vi "PersonnelFGV.vi"(7 "Actions":T1=enum."Read Personnel", 8 "error in (no error)":errorcluster, 9 "Data In":string, 10 "PUID":string) -> (0 "error out":errorcluster, 1 "Data Out":string)   [LabVIEW 2015]
uses:
  TypeDef/PersonnelActions.ctl
  TypeDef/PersonnelState.ctl
  LVClasses/Personnel/Personnel.lvclass
  LVClasses/Personnel/PersonnelType.ctl
  LVClasses/Personnel/Personnel.lvclass/Personnel.ctl
  LVClasses/Request/SummaryJsonCluster.ctl
  LVClasses/Personnel/Read Name.vi
  LVClasses/Personnel/Read Role.vi
  LVClasses/Personnel/Read UniqueID.vi
  LVClasses/Personnel/Read Requests.vi
  LVClasses/Personnel/Write Requests.vi
  LVClasses/Personnel/Write Name.vi
  LVClasses/Personnel/Write Role.vi
  LVClasses/Request/Request.lvclass
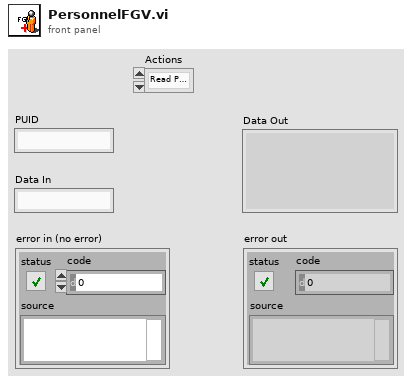
[diagram p1: front panel]
types:
  T1 = typedef "PersonnelActions.ctl" = enum16{"Init", "Read Personnel", "Add Personnel", "Remove Personnel", "Read Name", "Write Name", "Read Role", "Write Role", "Read Requests", "Add Requests", "Remove Requests", "Read PUIDs", "Read PUIDs for Role"}
  T2 = typedef "PersonnelState.ctl" = cluster{"Personnel":refnum<class "Personnel.lvclass">[]}
  T3 = typedef "Request.lvclass/SummaryJsonCluster.ctl" = cluster{"RequestID":string, "EnlapsedTime":i32, "Description":string, "Alarm":bool}
  T4 = typedef "Personnel.lvclass/PersonnelType.ctl" = enum16{"Nurse", "Doctor", "Cleanning", "Admin"}
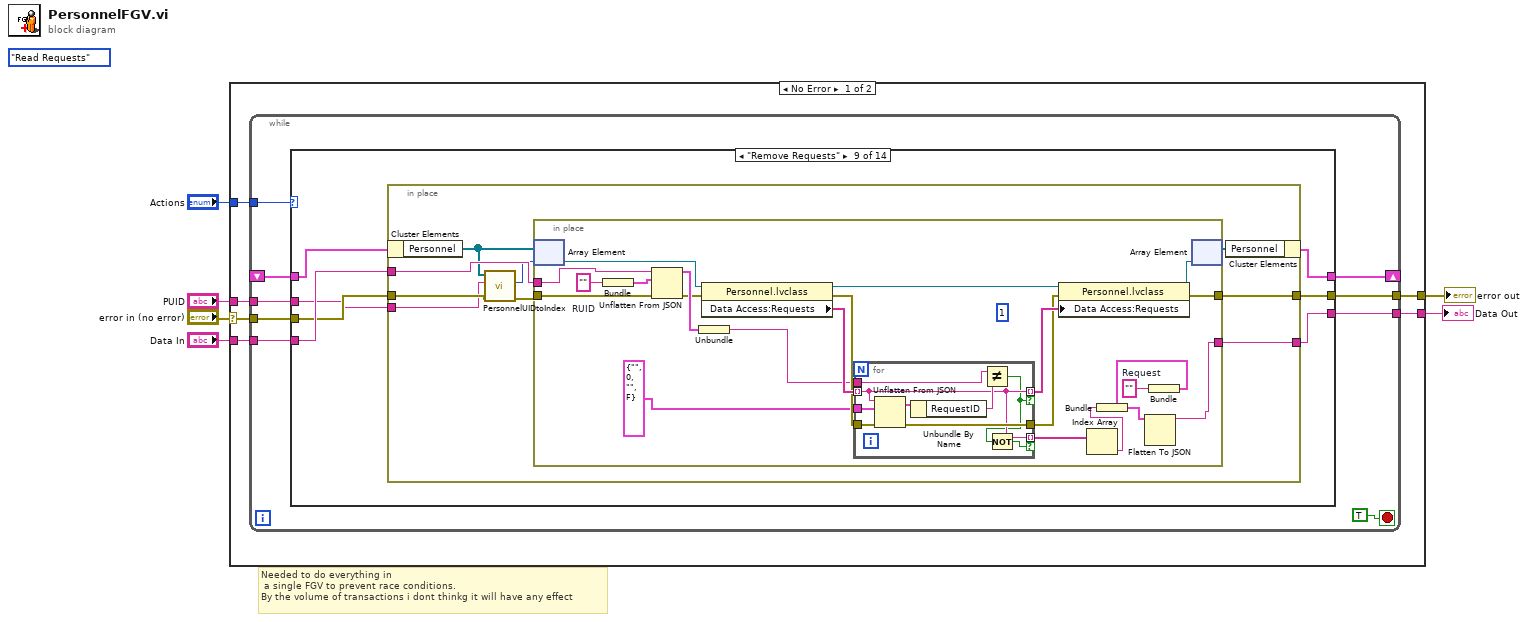
[diagram p0: block diagram]
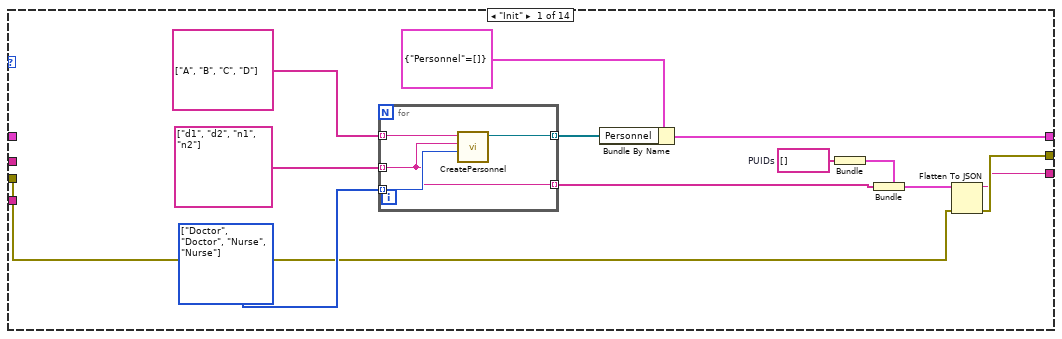
[diagram p2: hidden frame]
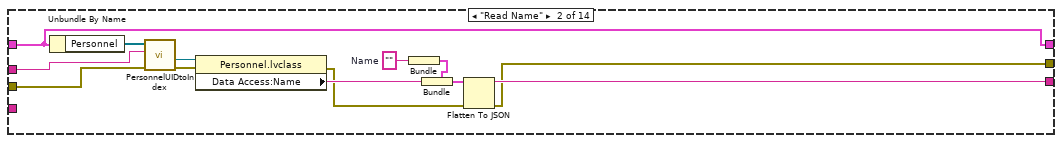
[diagram p3: hidden frame]
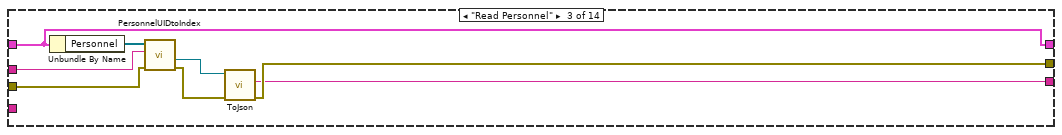
[diagram p4: hidden frame]
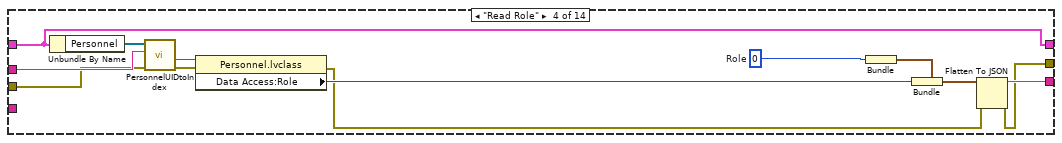
[diagram p5: hidden frame]
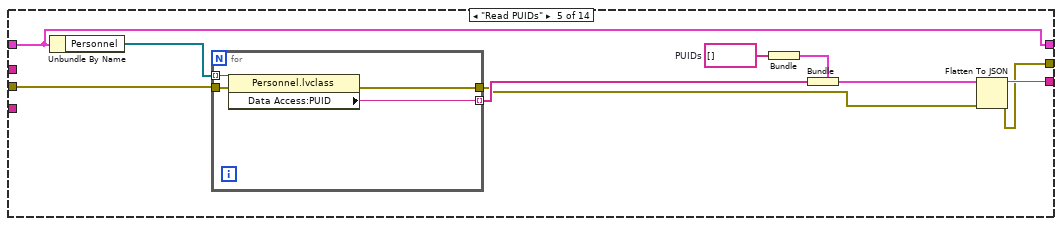
[diagram p6: hidden frame]
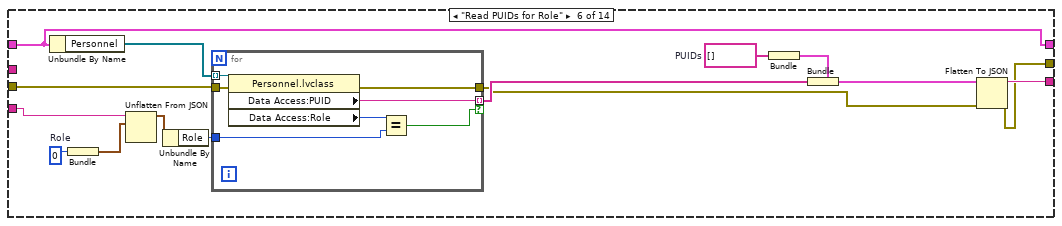
[diagram p7: hidden frame]
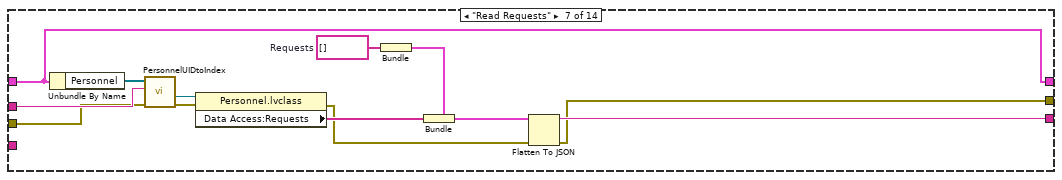
[diagram p8: hidden frame]
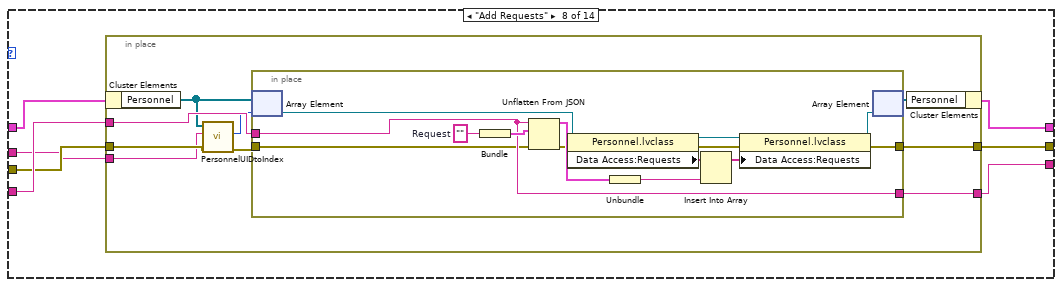
[diagram p9: hidden frame]
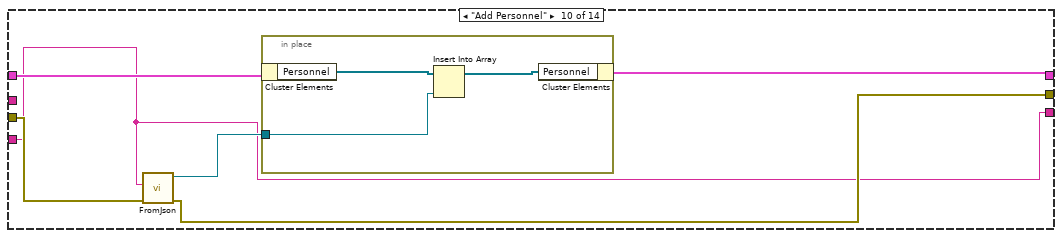
[diagram p10: hidden frame]
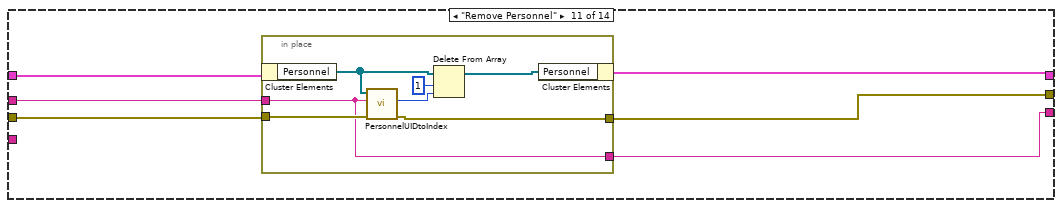
[diagram p11: hidden frame]
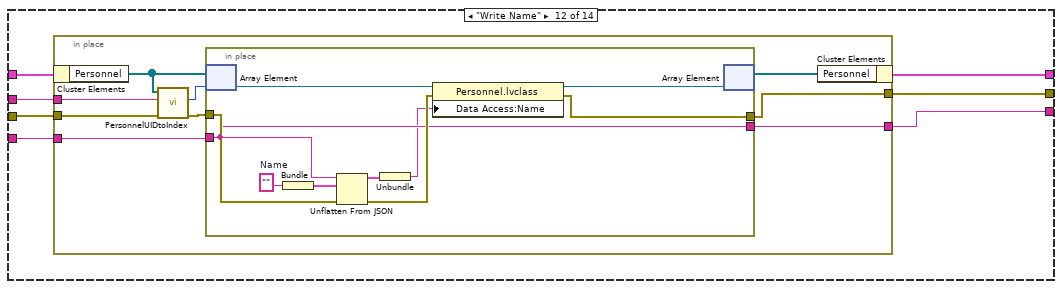
[diagram p12: hidden frame]
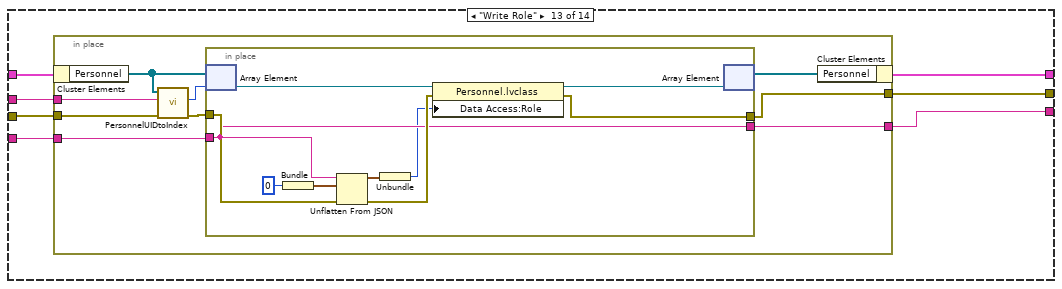
[diagram p13: hidden frame]
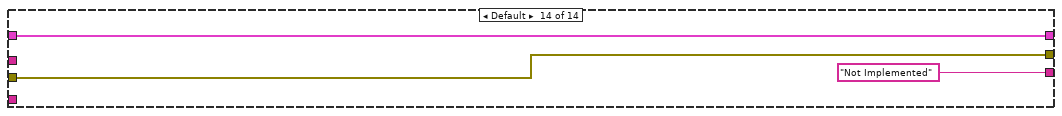
[diagram p14: hidden frame]
diagram:
  (unwired) PersonnelActions."Read Requests" ("Actions")
  # "Needed to do everything in\n a single FGV to prevent race conditions. \nBy the volume of transactions i dont thinkg it will have any effect"
  n1 = case shown="No Error" "error in (no error)" {
    selector: "error in (no error)" -> [w8 w276]
    tunnel: "Actions" -> [w12 _]
    tunnel: "PUID" -> [w11 _]
    tunnel: [w10 _] -> w4
    tunnel: "Data In" -> [w9 _]
    tunnel: [w7 w276] -> w1
    frame No Error {
      n2 = while {
        shift-right: [w19] -> _
        shift-left: _ -> [w18]
        tunnel: w12 -> [w20]
        tunnel: w11 -> [w17]
        tunnel: [w16] -> w10
        tunnel: w9 -> [w15]
        tunnel: w8 -> [w14]
        tunnel: [w13] -> w7
        stop <- TRUE ("stop") stop-if-true
        n3 = case shown="\"Remove Requests\"" w20 {
          tunnel: [w34 w51 w59 w72 w82 w101 w121 w123 w153 w200 w212 w226 w252 w275] -> w19
          tunnel: w18 -> [_ w51 w59 w72 w82 w101 w121 w128 w158 w204 w213 w227 w253 w275]
          tunnel: w17 -> [_ w49 w57 w70 _ _ w119 w124 w154 _ w209 w223 w249 _]
          tunnel: [w22 w45 w52 w66 w81 w100 w117 w122 w152 w199 w208 w221 w247 "Not Implemented" ("JSON string")] -> w16
          tunnel: w15 -> [_ _ _ _ _ w90 _ w127 w157 w199 _ w222 w248 _]
          tunnel: w14 -> [w25 w44 w56 w63 w74 w93 w112 w126 w156 w203 w211 w225 w251 w273]
          tunnel: [w26 w41 w53 w60 w80 w99 w109 w125 w155 w202 w210 w224 w250 w273] -> w13
          frame "Init" {
            w27 = string[] []  # PUIDs
            w31 = T4[] [enum."Doctor", enum."Doctor", enum."Nurse", enum."Nurse"] items=["Nurse", "Doctor", "Cleanning", "Admin"]
            n4 = for {
              tunnel: [w38] -> w32 mode=indexing
              tunnel: w31 -> [w37] mode=indexing
              tunnel: string[] ["d1", "d2", "n1", "n2"] -> [w35] mode=indexing
              tunnel: string[] ["A", "B", "C", "D"] -> [w36] mode=indexing
              tunnel: [w35] -> w23 mode=indexing
              n5 = call "CreatePersonnel.vi"("Role"=w37, "UniqueID"=w35, "Name"=w36) -> ("output cluster"=w38:refnum<class "Personnel.lvclass">)  [unwired: 7 in, 1 out]
            }
            n6 = Bundle By Name(cluster=T2 {"Personnel"=[]}, "Personnel"=w32) -> (w34:T2)
            n7 = Bundle("PUIDs"=w27) -> (w28:cluster{"PUIDs":string[]})  [unwired: 1 in]
            n8 = Bundle(cluster=w28, "PUIDs"=w23) -> (w24:cluster{"PUIDs":string[]})
            n9 = Flatten To JSON(anything=w24, error in (no error)=w25) -> (JSON string=w22:string, 11:w26:errorcluster)  [unwired: 1 in]
          }
          frame "Read Name" {
            w39 = ""  # Name
            n10 = Unbundle By Name(w51) -> ("Personnel"=w50:refnum<class "Personnel.lvclass">[])
            n11 = call "PersonnelUIDtoIndex.vi"("error in (no error)"=w44, "PUID"=w49, "Personnel in"=w50) -> ("error out"=w43:errorcluster, "Personnel"=w48:refnum<class "Personnel.lvclass">)  [unwired: 5 in, 2 out]
            n12 = property class="Personnel.lvclass"(reference=w48, error in=w43) -> (error out=w42:errorcluster, "Data Access:Name"=w47:string)  [unwired: 1 out]
            n13 = Bundle("Name"=w39) -> (w40:cluster{"Name":string})  [unwired: 1 in]
            n14 = Bundle(cluster=w40, "Name"=w47) -> (w46:cluster{"Name":string})
            n15 = Flatten To JSON(anything=w46, error in (no error)=w42) -> (JSON string=w45:string, 11:w41:errorcluster)  [unwired: 1 in]
          }
          frame "Read Personnel" {
            n16 = Unbundle By Name(w59) -> ("Personnel"=w58:refnum<class "Personnel.lvclass">[])
            n17 = call "PersonnelUIDtoIndex.vi"("error in (no error)"=w56, "PUID"=w57, "Personnel in"=w58) -> ("error out"=w55:errorcluster, "Personnel"=w54:refnum<class "Personnel.lvclass">)  [unwired: 5 in, 2 out]
            n18 = call "ToJson.vi"("error in (no error)"=w55, "Personnel in"=w54) -> ("error out"=w53:errorcluster, "PersonnelJson"=w52:string)  [unwired: 7 in, 1 out]
          }
          frame "Read Role" {
            w65 = 0  # Role
            n19 = Unbundle By Name(w72) -> ("Personnel"=w71:refnum<class "Personnel.lvclass">[])
            n20 = call "PersonnelUIDtoIndex.vi"("error in (no error)"=w63, "PUID"=w70, "Personnel in"=w71) -> ("error out"=w62:errorcluster, "Personnel"=w69:refnum<class "Personnel.lvclass">)  [unwired: 5 in, 2 out]
            n21 = property class="Personnel.lvclass"(reference=w69, error in=w62) -> (error out=w61:errorcluster, "Data Access:Role"=w68:T4)  [unwired: 1 out]
            n22 = Bundle("Role"=w65) -> (w64:cluster{"Role":i32})  [unwired: 1 in]
            n23 = Bundle(cluster=w64, "Role"=w68) -> (w67:cluster{"Role":i32})
            n24 = Flatten To JSON(anything=w67, error in (no error)=w61) -> (JSON string=w66:string, 11:w60:errorcluster)  [unwired: 1 in]
          }
          frame "Read PUIDs" {
            w77 = string[] []  # PUIDs
            n25 = Unbundle By Name(w82) -> ("Personnel"=w79:refnum<class "Personnel.lvclass">[])
            n26 = for {
              tunnel: w79 -> [w86] mode=indexing
              tunnel: [w85] -> w75 mode=indexing
              tunnel: w74 -> [w84]
              tunnel: [w83] -> w73
              n27 = property class="Personnel.lvclass"(reference=w86, error in=w84) -> (error out=w83:errorcluster, "Data Access:PUID"=w85:string)  [unwired: 1 out]
            }
            n28 = Bundle("PUIDs"=w77) -> (w78:cluster{"PUIDs":string[]})  [unwired: 1 in]
            n29 = Bundle(cluster=w78, "PUIDs"=w75) -> (w76:cluster{"PUIDs":string[]})
            n30 = Flatten To JSON(anything=w76, error in (no error)=w73) -> (JSON string=w81:string, 11:w80:errorcluster)  [unwired: 1 in]
          }
          frame "Read PUIDs for Role" {
            w91 = 0  # Role
            w96 = string[] []  # PUIDs
            n31 = Unbundle By Name(w101) -> ("Personnel"=w98:refnum<class "Personnel.lvclass">[])
            n32 = Bundle("Role"=w91) -> (w89:cluster{"Role":i32})  [unwired: 1 in]
            n33 = Unflatten From JSON(JSON string=w90, type and defaults=w89) -> (value=w88:cluster{"Role":i32})  [unwired: 5 in, 1 out]
            n34 = Unbundle By Name(w88) -> ("Role"=w87:i32)
            n35 = for {
              tunnel: w98 -> [w108] mode=indexing
              tunnel: [w107] -> w94 mode=indexing if=w102
              tunnel: w93 -> [w106]
              tunnel: [w105] -> w92
              tunnel: w87 -> [w103]
              n36 = property class="Personnel.lvclass"(reference=w108, error in=w106) -> (error out=w105:errorcluster, "Data Access:PUID"=w107:string, "Data Access:Role"=w104:T4)  [unwired: 1 out]
              n37 = Equal?(x=w104, y=w103) -> (x = y?=w102:bool)
            }
            n38 = Bundle("PUIDs"=w96) -> (w97:cluster{"PUIDs":string[]})  [unwired: 1 in]
            n39 = Bundle(cluster=w97, "PUIDs"=w94) -> (w95:cluster{"PUIDs":string[]})
            n40 = Flatten To JSON(anything=w95, error in (no error)=w92) -> (JSON string=w100:string, 11:w99:errorcluster)  [unwired: 1 in]
          }
          frame "Read Requests" {
            w115 = string[] []  # Requests
            n41 = Unbundle By Name(w121) -> ("Personnel"=w120:refnum<class "Personnel.lvclass">[])
            n42 = call "PersonnelUIDtoIndex.vi"("error in (no error)"=w112, "PUID"=w119, "Personnel in"=w120) -> ("error out"=w111:errorcluster, "Personnel"=w118:refnum<class "Personnel.lvclass">)  [unwired: 5 in, 2 out]
            n43 = property class="Personnel.lvclass"(reference=w118, error in=w111) -> (error out=w110:errorcluster, "Data Access:Requests"=w114:string[])  [unwired: 1 out]
            n44 = Bundle("Requests"=w115) -> (w116:cluster{"Requests":string[]})  [unwired: 1 in]
            n45 = Bundle(cluster=w116, "Requests"=w114) -> (w113:cluster{"Requests":string[]})
            n46 = Flatten To JSON(anything=w113, error in (no error)=w110) -> (JSON string=w117:string, 11:w109:errorcluster)  [unwired: 1 in]
          }
          frame "Add Requests" {
            n47 = in-place {
              in-place-border: [w135] -> w122
              in-place-border: w126 -> [w130]
              in-place-border: [w136] -> w125
              in-place-border: w127 -> [w134]
              in-place-border: w124 -> [w129]
              n48 = in-place-cluster #1(w128) -> ("Personnel"=w133:refnum<class "Personnel.lvclass">[])
              n49 = call "PersonnelUIDtoIndex.vi"("error in (no error)"=w130, "PUID"=w129, "Personnel in"=w133) -> ("error out"=w131:errorcluster, "Index"=w132:i32)  [unwired: 5 in, 2 out]
              n50 = in-place {
                in-place-border: w131 -> [w145]
                in-place-border: [w151] -> w136
                in-place-border: [w148] -> w135
                in-place-border: w134 -> [w148]
                w144 = ""  # Request
                n51 = in-place-array #2(w133, w132) -> (w146:refnum<class "Personnel.lvclass">)
                n52 = Bundle("Request"=w144) -> (w149:cluster{"Request":string})  [unwired: 1 in]
                n53 = Unflatten From JSON(JSON string=w148, type and defaults=w149, error in (no error)=w145) -> (value=w147:cluster{"Request":string}, error out=w142:errorcluster)  [unwired: 4 in]
                n54 = property class="Personnel.lvclass"(reference=w146, error in=w142) -> (reference out=w143:refnum<class "Personnel.lvclass">, error out=w141:errorcluster, "Data Access:Requests"=w140:string[])
                n55 = Unbundle(w147) -> ("Request"=w138:string)
                n56 = Insert Into Array(array=w140, new element=w138) -> (w139:string[])  [unwired: 1 in]
                n57 = property class="Personnel.lvclass"(reference=w143, error in=w141, "Data Access:Requests"=w139) -> (reference out=w150:refnum<class "Personnel.lvclass">, error out=w151:errorcluster)
                n58 = in-place-array #2(w150) -> (w137:refnum<class "Personnel.lvclass">[])  [unwired: 1 out]
              }
              n59 = in-place-cluster #1("Personnel"=w137) -> (w123:T2)
            }
          }
          frame "Remove Requests" {
            n60 = in-place {
              in-place-border: [w165] -> w152
              in-place-border: w156 -> [w160]
              in-place-border: [w166] -> w155
              in-place-border: w157 -> [w164]
              in-place-border: w154 -> [w159]
              n61 = in-place-cluster #3(w158) -> ("Personnel"=w163:refnum<class "Personnel.lvclass">[])
              n62 = call "PersonnelUIDtoIndex.vi"("error in (no error)"=w160, "PUID"=w159, "Personnel in"=w163) -> ("error out"=w161:errorcluster, "Index"=w162:i32)  [unwired: 5 in, 2 out]
              n63 = in-place {
                in-place-border: w161 -> [w183]
                in-place-border: [w189] -> w166
                in-place-border: [w168] -> w165
                in-place-border: w164 -> [w186]
                w172 = ""  # Request
                (unwired) 1 ("length")
                w182 = ""  # RUID
                n64 = in-place-array #4(w163, w162) -> (w184:refnum<class "Personnel.lvclass">)
                n65 = Bundle("RUID"=w182) -> (w187:cluster{"RUID":string})  [unwired: 1 in]
                n66 = Unflatten From JSON(JSON string=w186, type and defaults=w187, error in (no error)=w183) -> (value=w185:cluster{"RUID":string}, error out=w180:errorcluster)  [unwired: 4 in]
                n67 = Unbundle(w185) -> ("RUID"=w174:string)
                n68 = property class="Personnel.lvclass"(reference=w184, error in=w180) -> (reference out=w181:refnum<class "Personnel.lvclass">, error out=w177:errorcluster, "Data Access:Requests"=w179:string[])
                n69 = for {
                  tunnel: w179 -> [w192] mode=indexing
                  tunnel: [w192] -> w178 mode=indexing if=w190
                  tunnel: w177 -> [w198]
                  tunnel: [w197] -> w176
                  tunnel: T3 {"RequestID"="", "EnlapsedTime"=0, "Description"="", "Alarm"=FALSE} ("RequestTable") -> [w196]
                  tunnel: w174 -> [w193]
                  tunnel: [w192] -> w173 mode=indexing if=w191
                  n70 = Unflatten From JSON(JSON string=w192, type and defaults=w196, error in (no error)=w198) -> (value=w195:T3, error out=w197:errorcluster)  [unwired: 4 in]
                  n71 = Unbundle By Name(w195) -> ("RequestID"=w194:string)
                  n72 = Not Equal?(x=w193, y=w194) -> (x != y?=w190:bool)
                  n73 = Not(x=w190) -> (.not. x?=w191:bool)
                }
                n74 = property class="Personnel.lvclass"(reference=w181, error in=w176, "Data Access:Requests"=w178) -> (reference out=w188:refnum<class "Personnel.lvclass">, error out=w189:errorcluster)
                n75 = Index Array(array=w173) -> (element=w170:string)  [unwired: 1 in]
                n76 = Bundle("Request"=w172) -> (w171:cluster{"Request":string})  [unwired: 1 in]
                n77 = Bundle(cluster=w171, "Request"=w170) -> (w169:cluster{"Request":string})
                n78 = Flatten To JSON(anything=w169) -> (JSON string=w168:string)  [unwired: 2 in, 1 out]
                n79 = in-place-array #4(w188) -> (w167:refnum<class "Personnel.lvclass">[])  [unwired: 1 out]
              }
              n80 = in-place-cluster #3("Personnel"=w167) -> (w153:T2)
            }
          }
          frame "Add Personnel" {
            n81 = call "FromJson.vi"("error in (no error)"=w203, "PersonnelJson"=w199) -> ("error out"=w202:errorcluster, "Personnel out"=w201:refnum<class "Personnel.lvclass">)  [unwired: 8 in]
            n82 = in-place {
              in-place-border: w201 -> [w205]
              n83 = in-place-cluster #5(w204) -> ("Personnel"=w207:refnum<class "Personnel.lvclass">[])
              n84 = Insert Into Array(array=w207, new element=w205) -> (w206:refnum<class "Personnel.lvclass">[])  [unwired: 1 in]
              n85 = in-place-cluster #5("Personnel"=w206) -> (w200:T2)
            }
          }
          frame "Remove Personnel" {
            n86 = in-place {
              in-place-border: w209 -> [w214]
              in-place-border: w211 -> [w219]
              in-place-border: [w215] -> w210
              in-place-border: [w214] -> w208
              n87 = in-place-cluster #6(w213) -> ("Personnel"=w218:refnum<class "Personnel.lvclass">[])
              n88 = call "PersonnelUIDtoIndex.vi"("error in (no error)"=w219, "PUID"=w214, "Personnel in"=w218) -> ("error out"=w215:errorcluster, "Index"=w216:i32)  [unwired: 5 in, 2 out]
              n89 = Delete From Array(array=w218, length=1, index=w216) -> (array with subset deleted=w220:refnum<class "Personnel.lvclass">[])  [unwired: 1 out]
              n90 = in-place-cluster #6("Personnel"=w220) -> (w212:T2)
            }
          }
          frame "Write Name" {
            n91 = in-place {
              in-place-border: w223 -> [w236]
              in-place-border: w225 -> [w235]
              in-place-border: [w229] -> w224
              in-place-border: w222 -> [w231]
              in-place-border: [w228] -> w221
              n92 = in-place-cluster #7(w227) -> ("Personnel"=w234:refnum<class "Personnel.lvclass">[])
              n93 = call "PersonnelUIDtoIndex.vi"("error in (no error)"=w235, "PUID"=w236, "Personnel in"=w234) -> ("error out"=w230:errorcluster, "Index"=w232:i32)  [unwired: 5 in, 2 out]
              n94 = in-place {
                in-place-border: w231 -> [w241]
                in-place-border: w230 -> [w244]
                in-place-border: [w242] -> w229
                in-place-border: [w241] -> w228
                w240 = ""  # Name
                n95 = in-place-array #8(w234, w232) -> (w246:refnum<class "Personnel.lvclass">)
                n96 = Bundle("Name"=w240) -> (w239:cluster{"Name":string})  [unwired: 1 in]
                n97 = Unflatten From JSON(JSON string=w241, type and defaults=w239, error in (no error)=w244) -> (value=w238:cluster{"Name":string}, error out=w243:errorcluster)  [unwired: 4 in]
                n98 = Unbundle(w238) -> ("Name"=w237:string)
                n99 = property class="Personnel.lvclass"(reference=w246, error in=w243, "Data Access:Name"=w237) -> (reference out=w245:refnum<class "Personnel.lvclass">, error out=w242:errorcluster)
                n100 = in-place-array #8(w245) -> (w233:refnum<class "Personnel.lvclass">[])  [unwired: 1 out]
              }
              n101 = in-place-cluster #7("Personnel"=w233) -> (w226:T2)
            }
          }
          frame "Write Role" {
            n102 = in-place {
              in-place-border: w249 -> [w262]
              in-place-border: w251 -> [w261]
              in-place-border: [w255] -> w250
              in-place-border: w248 -> [w257]
              in-place-border: [w254] -> w247
              n103 = in-place-cluster #9(w253) -> ("Personnel"=w260:refnum<class "Personnel.lvclass">[])
              n104 = call "PersonnelUIDtoIndex.vi"("error in (no error)"=w261, "PUID"=w262, "Personnel in"=w260) -> ("error out"=w256:errorcluster, "Index"=w258:i32)  [unwired: 5 in, 2 out]
              n105 = in-place {
                in-place-border: w257 -> [w267]
                in-place-border: w256 -> [w270]
                in-place-border: [w268] -> w255
                in-place-border: [w267] -> w254
                n106 = in-place-array #10(w260, w258) -> (w272:refnum<class "Personnel.lvclass">)
                n107 = Bundle("Role"=0) -> (w266:cluster{"Role":i32})  [unwired: 1 in]
                n108 = Unflatten From JSON(JSON string=w267, type and defaults=w266, error in (no error)=w270) -> (value=w265:cluster{"Role":i32}, error out=w269:errorcluster)  [unwired: 4 in]
                n109 = Unbundle(w265) -> ("Role"=w264:i32)
                n110 = property class="Personnel.lvclass"(reference=w272, error in=w269, "Data Access:Role"=w264) -> (reference out=w271:refnum<class "Personnel.lvclass">, error out=w268:errorcluster)
                n111 = in-place-array #10(w271) -> (w259:refnum<class "Personnel.lvclass">[])  [unwired: 1 out]
              }
              n112 = in-place-cluster #9("Personnel"=w259) -> (w252:T2)
            }
          }
          frame Default {
          }
        }
      }
    }
    frame Error {
    }
  }
  "Data Out" <- w4
  "error out" <- w1
